vi "Read Valid Messages.vi"(8 "error in (no error)":errorcluster, 11 "Passive Hardware in":refnum<class "Passive Hardware.lvclass">) -> (0 "error out":errorcluster, 2 "Valid Messages":string[](array[string]), 3 "Passive Hardware out":refnum<class "Passive Hardware.lvclass">)   [LabVIEW 2020, in "RxnRover.lvlib" / "Passive Hardware.lvclass"]
uses:
  Passive Hardware.lvclass
  Passive Hardware.lvclass/Passive Hardware.ctl
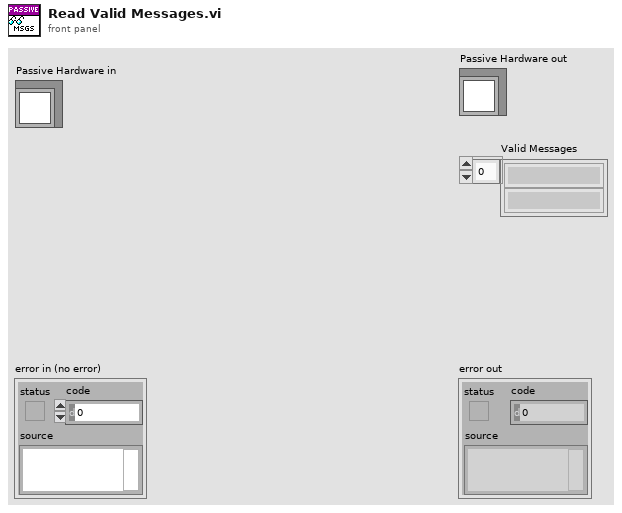
[diagram p1: front panel]
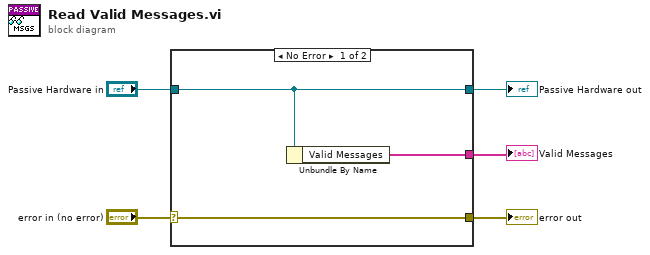
[diagram p0: block diagram]
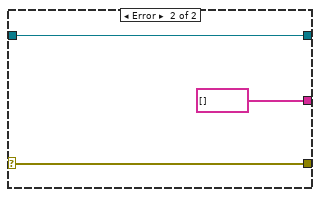
[diagram p2: hidden frame]
diagram:
  n1 = case shown="No Error" "error in (no error)" {
    selector: "error in (no error)" -> [w6 w11]
    tunnel: "Passive Hardware in" -> [w7 w10]
    tunnel: [w8 string[] []] -> w1
    tunnel: [w7 w10] -> w4
    tunnel: [w6 w11] -> w3
    frame No Error {
      n2 = Unbundle By Name(w7) -> ("Valid Messages"=w8:string[])
    }
    frame Error {
    }
  }
  "error out" <- w3
  "Passive Hardware out" <- w4
  "Valid Messages" <- w1
